vi "GetDeleteChannel_CLK.vi"(7 "CHANNEL":string[][](array[string]), 10 "CtlRef":refnum<vi>) -> (1 "Finded":bool, 2 "通道":string[](array[string]))   [LabVIEW 2015]
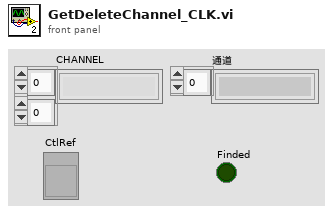
[diagram p1: front panel]
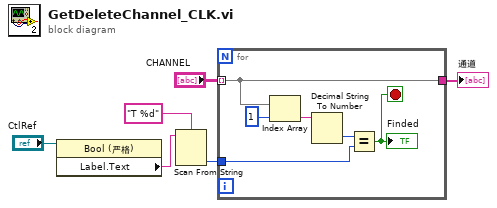
[diagram p0: block diagram]
diagram:
  n1 = property class="Bool (严格)"(reference="CtlRef") -> ("Label.Text"=w4:string)  [unwired: 1 in, 2 out]
  n2 = Scan From String(format string="T %d", input string=w4) -> (output 1=w1:i32)  [unwired: 3 in, 3 out]
  n3 = for {
    tunnel: "CHANNEL" -> [w12] mode=indexing
    tunnel: [w12] -> w2
    tunnel: w1 -> [w8]
    stop <- w7 stop-if-true
    n4 = Index Array(array=w12, index=1) -> (element=w10:string)
    n5 = Decimal String To Number(string=w10) -> (number=w9:i32)  [unwired: 2 in, 1 out]
    n6 = Equal?(x=w9, y=w8) -> (x = y?=w7:bool)
    "Finded" <- w7
  }
  "通道" <- w2
